vi "GetFPOwnerType.vi"(7 "PythonConverter_GUI in":refnum<class "PythonConverter_GUI.lvclass">, 8 "error in":errorcluster, 11 "Object in":refnum<class "GObject.lvclass">) -> (0 "error out":errorcluster, 3 "Object out":refnum<class "GObject.lvclass">, 4 "owner":T1, 5 "PythonConverter_GUI out":refnum<class "PythonConverter_GUI.lvclass">)   [LabVIEW 2014, in "Raspberry Pi Compatible Compiler for LabVIEW.lvlib" / "PythonConverter_GUI.lvclass"]
uses:
  PythonConverter_GUI.lvclass
  VI Interpreter/Classes/GObject/GObject.lvclass
  TypeDefs/FPOwnerClassTD.ctl
  PythonConverter_GUI.lvclass/PythonConverter_GUI.ctl
  VI Interpreter/Classes/Generic/Generic.lvclass/Generic.ctl
  VI Interpreter/Classes/VI Interpreter/VI Interpreter.lvclass
  VI Interpreter/Classes/Generic/Generic.lvclass
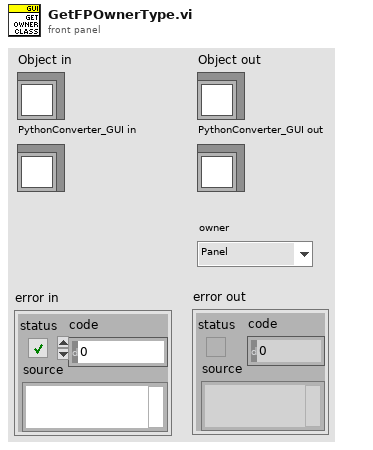
[diagram p1: front panel]
types:
  T1 = typedef "Raspberry Pi Compatible Compiler for LabVIEW.lvlib/PythonConverter_GUI.lvclass/FPOwnerClassTD.ctl" = enum16{"Panel", "Array", "Cluster", "Tab control"}
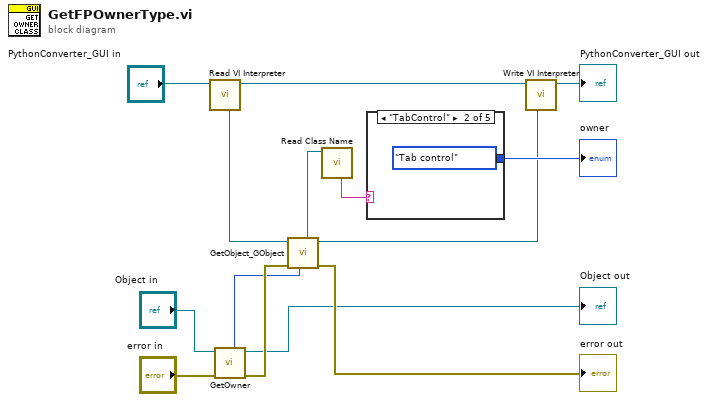
[diagram p0: block diagram]
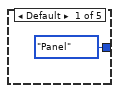
[diagram p2: hidden frame]
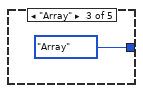
[diagram p3: hidden frame]
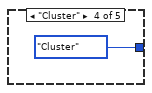
[diagram p4: hidden frame]
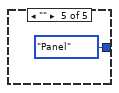
[diagram p5: hidden frame]
diagram:
  n1 = call "Read VI Interpreter.vi"("PythonConverter_GUI in"="PythonConverter_GUI in") -> ("PythonConverter_GUI out"=w3:refnum<class "PythonConverter_GUI.lvclass">, "VI Interpreter"=w4:refnum<class "VI Interpreter.lvclass">)  [unwired: 7 in]
  n2 = call-dynamic "GetOwner.vi"("error in"="error in", "GObject in"="Object in") -> ("error out"=w12:errorcluster, "GObject out"=→"Object out":refnum<class "GObject.lvclass">, "Owner"=w9:i32)  [unwired: 5 in]
  n3 = call "GetObject_GObject.vi"("UID"=w9, "error in"=w12, "VI Interpreter in"=w4) -> ("error out"=→"error out":errorcluster, "VI Interpreter out"=w1:refnum<class "VI Interpreter.lvclass">, "GObject"=w11:refnum<class "GObject.lvclass">)  [unwired: 3 in, 1 out]
  n4 = call "Read Class Name.vi"("Generic in"=w11) -> ("Class Name"=w10:string)  [unwired: 7 in, 1 out]
  n5 = case shown="\"TabControl\"" w10 {
    tunnel: [FPOwnerClassTD."Panel" ("owner") FPOwnerClassTD."Tab control" ("owner") FPOwnerClassTD."Array" ("owner") FPOwnerClassTD."Cluster" ("owner") FPOwnerClassTD."Panel" ("owner")] -> w8
    frame Default {
    }
    frame "TabControl" {
    }
    frame "Array" {
    }
    frame "Cluster" {
    }
    frame "" {
    }
  }
  "owner" <- w8
  n6 = call "Write VI Interpreter.vi"("VI Interpreter"=w1, "PythonConverter_GUI in"=w3) -> ("PythonConverter_GUI out"=→"PythonConverter_GUI out":refnum<class "PythonConverter_GUI.lvclass">)  [unwired: 7 in]
